vi "depth read.vi"(1 "Increment Button":bool, 2 "Read String Pot":bool=TRUE, 3 "Initialize Debug":bool, 4 "Debug":bool) -> (0 "Distance":dbl format="%.2f")   [LabVIEW 2016]
uses:
  ad interface/Global_SIM_switch.vi
  Kpro Globals.vi
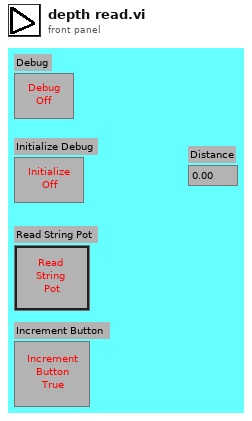
[diagram p1: front panel]
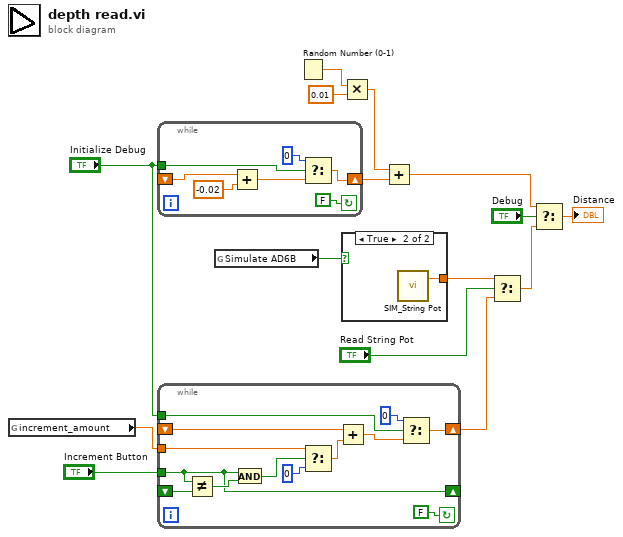
[diagram p0: block diagram]
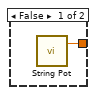
[diagram p2: hidden frame]
diagram:
  n1 = global read "Kpro Globals.vi" "increment_amount"() -> (w1:dbl)
  n2 = while {
    tunnel: "Initialize Debug" -> [w21]
    shift-left: _ -> [w19]
    shift-right: [w20] -> w13
    stop <- FALSE continue-if-true
    n3 = Add(x=w19, y=-0.02) -> (x+y=w17:dbl)
    n4 = Select(t=0, s=w21, f=w17) -> (s? t:f=w20:dbl)
  }
  n5 = while {
    tunnel: w1 -> [w23]
    tunnel: "Increment Button" -> [w25]
    shift-left: _ -> [w30]
    shift-right: [w25] -> _
    tunnel: "Initialize Debug" -> [w31]
    shift-left: _ -> [w33]
    shift-right: [w34] -> w4
    stop <- FALSE continue-if-true
    n6 = Not Equal?(x=w25, y=w30) -> (x != y?=w28:bool)
    n7 = And(x=w25, y=w28) -> (x .and. y?=w26:bool)
    n8 = Select(t=w23, s=w26, f=0) -> (s? t:f=w29:dbl)
    n9 = Add(x=w33, y=w29) -> (x+y=w32:dbl)
    n10 = Select(t=0, s=w31, f=w32) -> (s? t:f=w34:dbl)
  }
  n11 = global read "Global_SIM_switch.vi" "Simulate AD6B"() -> (w2:bool)
  n12 = Random Number (0-1)() -> (number: 0 to 1=w15:dbl)
  n13 = Multiply(x=w15, y=0.01) -> (x*y=w12:dbl)
  n14 = case shown="True" w2 {
    tunnel: [w36 w37] -> w3
    frame False {
      n15 = call "String Pot.vi"() -> ("Distance (in)"=w36:dbl)  [unwired: 3 in]
    }
    frame True {
      n16 = call "SIM_String Pot.vi"() -> ("Distance (in)"=w37:dbl)  [unwired: 3 in]
    }
  }
  n17 = Add(x=w12, y=w13) -> (x+y=w9:dbl)
  n18 = Select(t=w3, s="Read String Pot", f=w4) -> (s? t:f=w8:dbl)
  n19 = Select(t=w9, s="Debug", f=w8) -> (s? t:f=→"Distance":dbl)
